vi "Checa destino cupula.vi"(6 "ErroCupCustom":i16, 9 "Target":u16) -> (1 "angCUP":string, 2 "moverCup":bool, 3 "angTarget":string)   [LabVIEW 2018]
uses:
  Global_Telescopio.vi
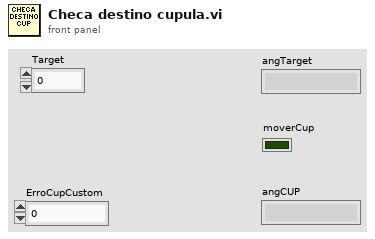
[diagram p1: front panel]
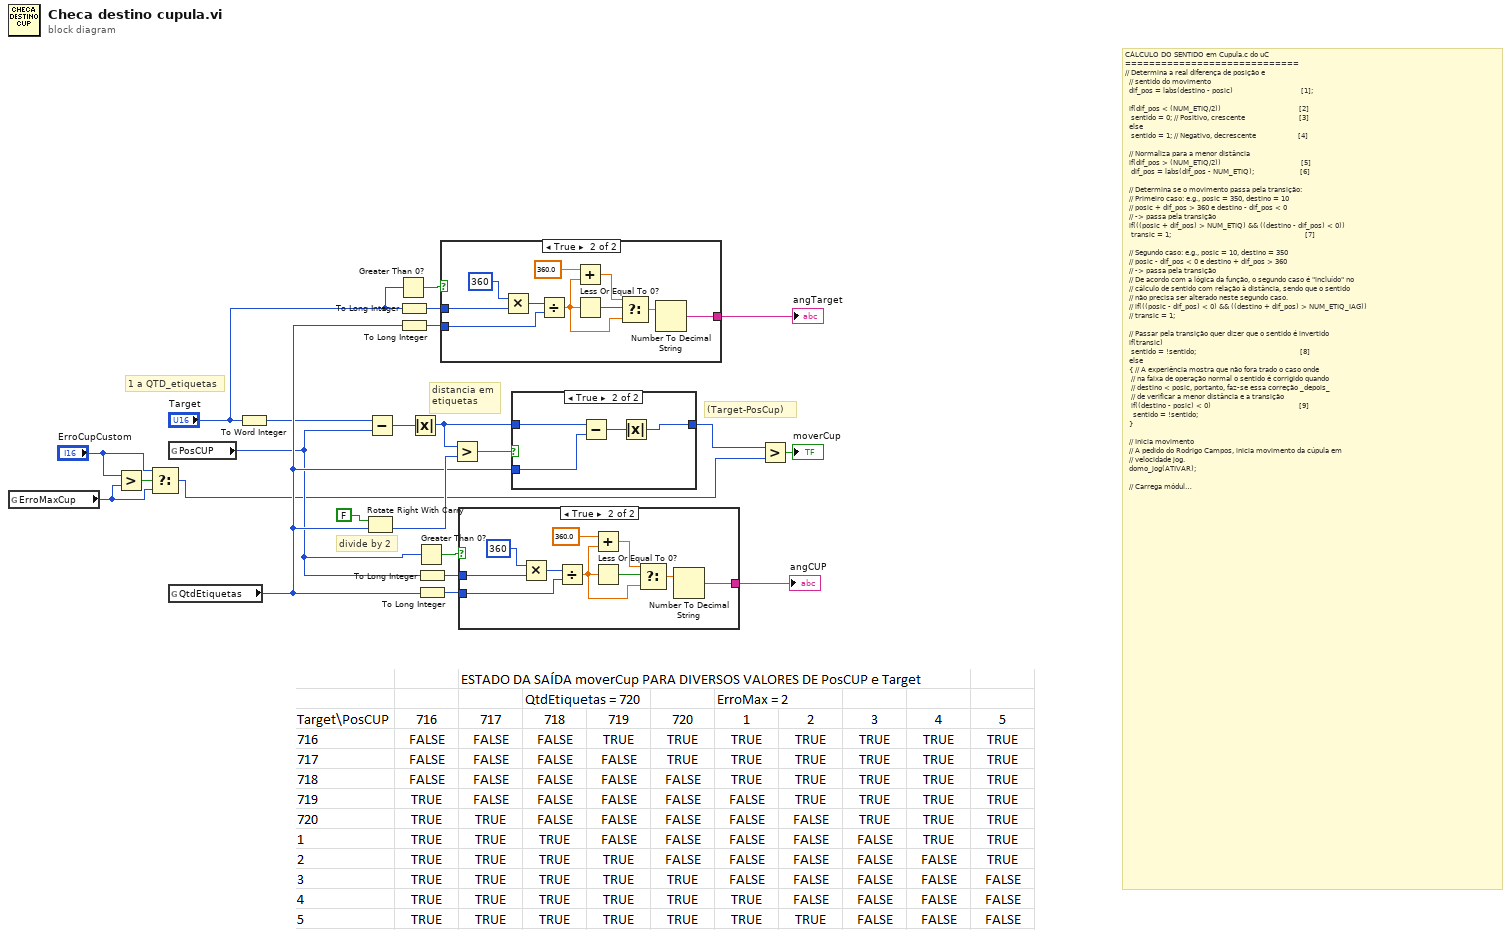
[diagram p0: block diagram]
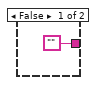
[diagram p2: hidden frame]
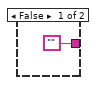
[diagram p3: hidden frame]
diagram:
  # "(Target-PosCup)"
  # "CÁLCULO DO SENTIDO em Cupula.c do uC\n=============================\t\t\n// Determina a real diferença de posição e\n\t\t// sentido do movimento\n\t\tdif_pos = labs(destino - posic)                                  [1];\n\n\t\tif(dif_pos < (NUM_ETIQ/2))                                       [2]\n\t\t\tsentido = 0;\t// Positivo, crescente                           [3]\n\t\telse\n\t\t\tsentido = 1;\t// Negativo, decrescente                     [4]\n\t\n\t\t// Normaliza para a menor distância\n\t\tif(dif_pos > (NUM_ETIQ/2))                                        [5]\n\t\t\tdif_pos = labs(dif_pos - NUM_ETIQ);                       [6]\n\n\t\t// Determina se o movimento passa pela transição:\n\t\t// Primeiro caso: e.g., posic = 350, destino = 10\n\t\t// posic + dif_pos > 360 e destino - dif_pos < 0 \n\t\t// -> passa pela transição\n\t\tif(((posic + dif_pos) > NUM_ETIQ) && ((destino - dif_pos) < 0))\n\t\t\ttransic = 1;                                                                   [7]\n\n\t\t// Segundo caso: e.g., posic = 10, destino = 350\n\t\t// posic - dif_pos < 0 e destino + dif_pos > 360\n\t\t// -> passa pela transição\n\t\t// De acordo com a lógica da função, o segundo caso é \"incluído\" no\n\t\t// cálculo de sentido com relação à distância, sendo que o sentido\n\t\t// não precisa ser alterado neste segundo caso.\n\t\t// if(((posic - dif_pos) < 0) && ((destino + dif_pos) > NUM_ETIQ_IAG))\n\t\t//\ttransic = 1;\n\n\t\t// Passar pela transição quer dizer que o sentido é invertido\n\t\tif(transic)\n\t\t\tsentido = !sentido;                                                    [8]\n\t\telse\n\t\t{\t// A experiência mostra que não fora trado o caso onde\n\t\t\t// na faixa de operação normal o sentido é corrigido quando\n\t\t\t// destino < posic, portanto, faz-se essa correção _depois_\n\t\t\t// de verificar a menor distância e a transição\n\t\t\tif((destino - posic) < 0)                                            [9]\n\t\t\t\tsentido = !sentido;\n\t\t}\n\n\t\t// Inicia movimento\n\t\t// A pedido do Rodrigo Campos, inicia movimento da cúpula em\n\t\t// velocidade jog.\n\t\tdomo_jog(ATIVAR);\n\n\t\t// Carrega módulo TIMEOUT1 com 4s.\n\t\tset_timeout(1,200,1);\n\n\t\tif(!sentido)\n\t\t\tdomo_pos(ATIVAR);\n\t\telse\n\t\t\tdomo_neg(ATIVAR);"
  # "divide by 2"
  # "1 a QTD_etiquetas"
  # "distancia em\netiquetas"
  n1 = global read "Global_Telescopio.vi" "ErroMaxCup"() -> (w2:i16)
  n2 = Greater?(x="ErroCupCustom", y=w2) -> (0:w4:bool)
  n3 = Select(t="ErroCupCustom", s=w4, f=w2) -> (s? t:f=w1:i16)
  n4 = global read "Global_Telescopio.vi" "PosCUP"() -> (w5:i16)
  n5 = global read "Global_Telescopio.vi" "QtdEtiquetas"() -> (w7:i16)
  n6 = To Word Integer(number="Target") -> (16bit integer=w6:i16)
  n7 = Rotate Right With Carry(2:w7, 3:FALSE ("carry")) -> (0:w16:i16)  [unwired: 1 out]
  n8 = Subtract(x=w6, y=w5) -> (x-y=w19:i16)
  n9 = Greater Than 0?(x="Target") -> (x > 0?=w10:bool)
  n10 = To Long Integer(number="Target") -> (32bit integer=w12:i32)
  n11 = To Long Integer(number=w7) -> (32bit integer=w11:i32)
  n12 = Absolute Value(x=w19) -> (abs(x)=w22:i16)
  n13 = Greater Than 0?(x=w5) -> (x > 0?=w15:bool)
  n14 = To Long Integer(number=w5) -> (32bit integer=w13:i32)
  n15 = To Long Integer(number=w7) -> (32bit integer=w14:i32)
  n16 = case shown="True" w10 {
    tunnel: ["" w33] -> w9
    tunnel: w11 -> [_ w26]
    tunnel: w12 -> [_ w25]
    frame False {
    }
    frame True {
      n17 = Multiply(x=360, y=w25) -> (x*y=w32:i32)
      n18 = Divide(x=w32, y=w26) -> (x/y=w29:dbl)
      n19 = Add(x=360.0, y=w29) -> (x+y=w27:dbl)
      n20 = Less Or Equal To 0?(x=w29) -> (x <= 0?=w31:bool)
      n21 = Select(t=w27, s=w31, f=w29) -> (s? t:f=w30:dbl)
      n22 = Number To Decimal String(number=w30) -> (decimal integer string=w33:string)  [unwired: 1 in]
    }
  }
  "angTarget" <- w9
  n23 = Greater?(x=w22, y=w16) -> (0:w23:bool)
  n24 = case shown="True" w15 {
    tunnel: ["" w44] -> w18
    tunnel: w14 -> [_ w37]
    tunnel: w13 -> [_ w36]
    frame False {
    }
    frame True {
      n25 = Multiply(x=360, y=w36) -> (x*y=w43:i32)
      n26 = Divide(x=w43, y=w37) -> (x/y=w40:dbl)
      n27 = Add(x=360.0, y=w40) -> (x+y=w38:dbl)
      n28 = Less Or Equal To 0?(x=w40) -> (x <= 0?=w42:bool)
      n29 = Select(t=w38, s=w42, f=w40) -> (s? t:f=w41:dbl)
      n30 = Number To Decimal String(number=w41) -> (decimal integer string=w44:string)  [unwired: 1 in]
    }
  }
  "angCUP" <- w18
  n31 = case shown="True" w23 {
    tunnel: w22 -> [w46 w50]
    tunnel: [w46 w48] -> w21
    tunnel: w7 -> [_ w47]
    frame False {
    }
    frame True {
      n32 = Subtract(x=w50, y=w47) -> (x-y=w49:i16)
      n33 = Absolute Value(x=w49) -> (abs(x)=w48:i16)
    }
  }
  n34 = Greater?(x=w21, y=w1) -> (0:→"moverCup":bool)
